vi "Configure Delay.vi"(7 "Config.Model":T1, 8 "error in (no error)":errorcluster, 9 "Horizontal Delay (0 s)":dbl, 10 "Enable Delay (T: Enable)":bool=TRUE, 11 "VISA resource name":refnum<visa-resource-name>) -> (0 "error out":errorcluster, 3 "VISA resource name out":refnum<visa-resource-name>)   [LabVIEW 2017, in "Scope.lvlib"]
doc: "Configures the horizontal delay settings."
uses:
  Scope.lvlib
  Controls/Models.ctl
  Third Party Drivers/Tektronix DPO MSO 2000 4000 Series/Tektronix DPO MSO 2000 4000 Series.lvlib
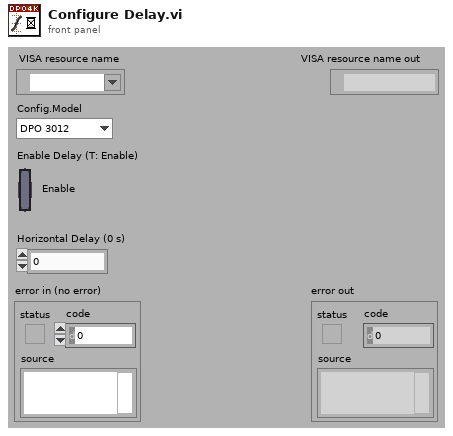
[diagram p1: front panel]
types:
  T1 = typedef "Scope.lvlib/Models.ctl" = enum16{"DPO 3012", "DPO 2012B", "TDS 3012C"}
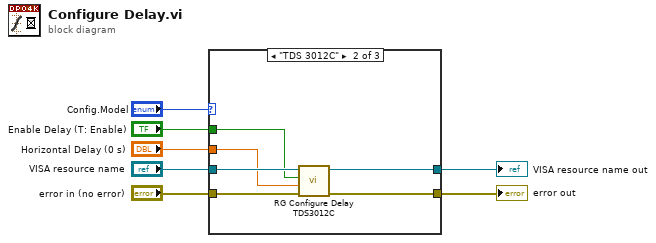
[diagram p0: block diagram]
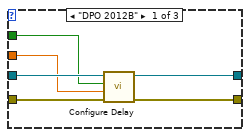
[diagram p2: hidden frame]
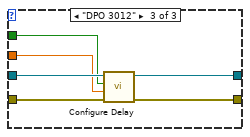
[diagram p3: hidden frame]
diagram:
  n1 = case shown="\"TDS 3012C\"" "Config.Model" {
    tunnel: "error in (no error)" -> [w13 w19 w25]
    tunnel: [w12 w18 w24] -> w6
    tunnel: "VISA resource name" -> [w11 w17 w23]
    tunnel: [w10 w16 w22] -> w4
    tunnel: "Enable Delay (T: Enable)" -> [w8 w15 w21]
    tunnel: "Horizontal Delay (0 s)" -> [w9 w14 w20]
    frame "DPO 2012B" {
      n2 = call "Configure Delay.vi"("error in (no error)"=w13, "Horizontal Delay (0 s)"=w9, "Enable Delay (T: Enable)"=w8, "VISA resource name"=w11) -> ("error out"=w12:errorcluster, "VISA resource name out"=w10:refnum<visa-resource-name>)  [unwired: 6 in]
    }
    frame "TDS 3012C" {
      n3 = call "RG Configure Delay TDS3012C.vi"("error in (no error)"=w19, "Horizontal Delay (0 s)"=w14, "Enable Delay (T: Enable)"=w15, "VISA resource name"=w17) -> ("error out"=w18:errorcluster, "VISA resource name out"=w16:refnum<visa-resource-name>)  [unwired: 6 in]
    }
    frame "DPO 3012" {
      n4 = call "Configure Delay.vi"("error in (no error)"=w25, "Horizontal Delay (0 s)"=w20, "Enable Delay (T: Enable)"=w21, "VISA resource name"=w23) -> ("error out"=w24:errorcluster, "VISA resource name out"=w22:refnum<visa-resource-name>)  [unwired: 6 in]
    }
  }
  "error out" <- w6
  "VISA resource name out" <- w4
